vi "asdasd.vi"(0 "Device":u32, 1 "Duration (s)":dbl=1.0, 2 "Sample rate (Hz)":dbl=44100.0, 3 "#Channels":i32=1, 4 "Resolution (bits)":i32=16, 5 "error in (no error)":errorcluster) -> (14 "Data":dynamicdata(graph), 19 "error out":errorcluster)   [LabVIEW 2019]
doc: "Acquires data from a sound device. This Express VI automatically configures an input task, acquires the data, and clears the task after the acquisition completes.\n--------------------\n\nThis Express VI is configured as follows:\n\nDevice: 0\nDuration: 1 s\nSample rate: 44100 Hz\n# Channels: 1\nResolution: 16 bits"
panel:
  in  "Path":path
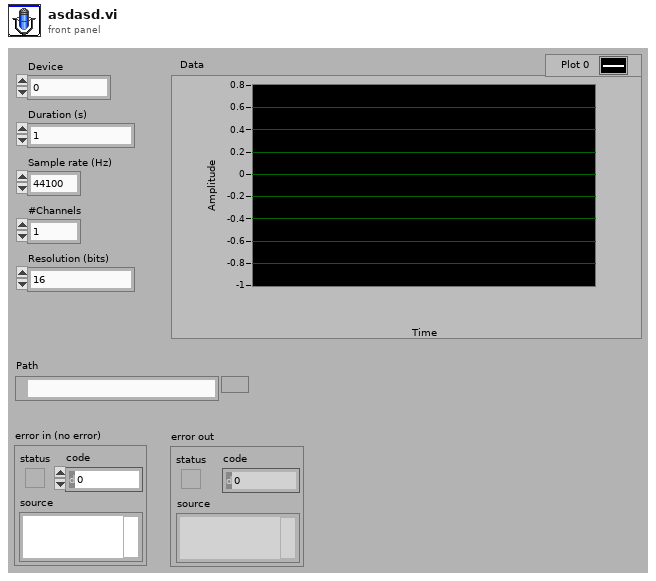
[diagram p1: front panel]
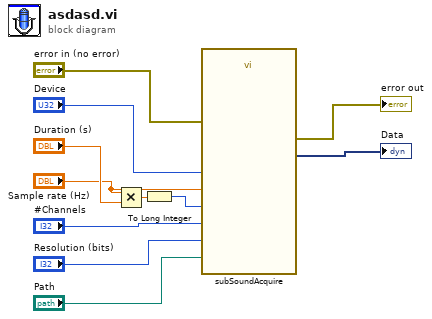
[diagram p0: block diagram]
diagram:
  n1 = Multiply(x="Sample rate (Hz)", y="Duration (s)") -> (x*y=w7:dbl)
  n2 = To Long Integer(number=w7) -> (32bit integer=w6:i32)
  n3 = call <vilib>:"subSoundAcquire.vi"("Device"="Device", "Resolution (bits)"="Resolution (bits)", "Sample rate (Hz)"="Sample rate (Hz)", "Samples per channel"=w6, "#Channels"="#Channels", "error in (no error)"="error in (no error)", "Path"="Path") -> ("Data"=→"Data":dynamicdata, "error out"=→"error out":errorcluster)  [unwired: 11 in]
